vi "Configure Multi Eval Meas Limit OBW.vi"(6 "Limit OBW (40e6)":dbl=40000000.0 format="%^.3e", 7 "Limit OBW Enabled (Value)":i32(ring)=2 items=["Off", "On", "Value"], 8 "error in (no error)":errorcluster, 9 "Bandwidth (5 MHz)":T1=5 items=["5 MHz"=5, "10 MHz"=10, "15 MHz"=15, "20 MHz"=20, "25 MHz"=25, "30 MHz"=30, "40 MHz"=40, "50 MHz"=50, "60 MHz"=60, "80 MHz"=80, "90 MHz"=90, "100 MHz"=100], 10 "Instance (1)":T2=1, 11 "VISA resource name":refnum<visa-resource-name>) -> (0 "error out":errorcluster, 3 "VISA resource name out":refnum<visa-resource-name>)   [LabVIEW 2020, in "Rohde&Schwarz CMWXP NR FR1 Measurement.lvlib"]
doc: "Defines an upper limit for the occupied bandwidth, depending on the channel bandwidth (for NR SA).\n\nAttributes:\nRSCMWXPNRFR1M_ATTR_MULTI_EVAL_MEAS_LIMIT_OBW_ENABLED\nRSCMWXPNRFR1M_ATTR_MULTI_EVAL_MEAS_LIMIT_OBW\n\nRemote-control command:\nCONFigure:NRSub:MEAS<i>:MEValuation:LIMit:SEMask:OBWLimit:CBANdwidth<bw>"
uses:
  <instrlib>/Rohde&Schwarz CMWXP NR FR1 Measurement/Rohde&Schwarz CMWXP NR FR1 Measurement.lvlib
  <instrlib>/Rohde&Schwarz CMWXP NR FR1 Measurement/Private/_Instance.ctl
  <instrlib>/Rohde&Schwarz CMWXP NR FR1 Measurement/Private/_Bandwidth.ctl
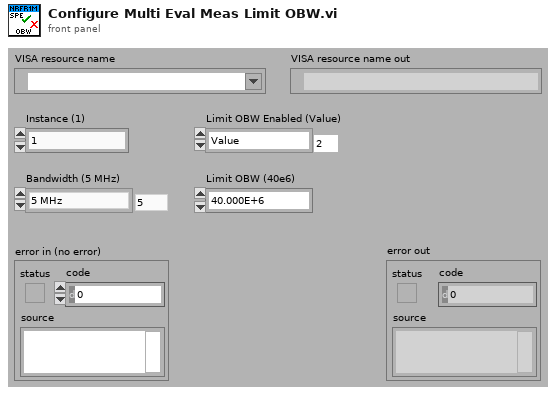
[diagram p1: front panel]
types:
  T1 = typedef "Rohde&Schwarz CMWXP NR FR1 Measurement.lvlib/_Bandwidth.ctl" = i32
  T2 = typedef "Rohde&Schwarz CMWXP NR FR1 Measurement.lvlib/_Instance.ctl" = i32
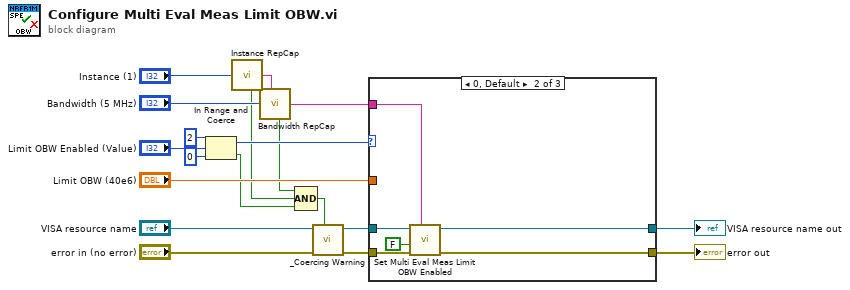
[diagram p0: block diagram]
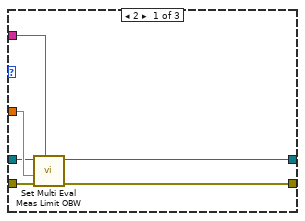
[diagram p2: hidden frame]
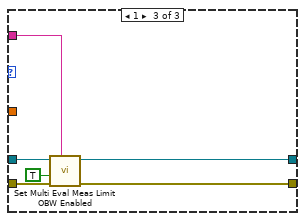
[diagram p3: hidden frame]
diagram:
  n1 = In Range and Coerce(upper limit=2, x="Limit OBW Enabled (Value)", lower limit=0) -> (coerced(x)=w5:i32, In Range?=w4:bool)
  n2 = call <instrlib>:"Instance RepCap.vi"("Instance In"="Instance (1)") -> ("In Range?"=w2:bool, "RepCap Identifier Out"=w15:string)  [unwired: 1 in]
  n3 = call <instrlib>:"Bandwidth RepCap.vi"("Bandwidth (5 MHz)"="Bandwidth (5 MHz)", "RepCap String In (\"\")"=w15) -> ("In Range?"=w3:bool, "RepCap Identifier Out"=w9:string)
  n4 = Compound Arithmetic op=AND(w3, w2, w4) -> (w1:bool)
  n5 = call <instrlib>:"_Coercing Warning.vi"("In Range?"=w1, "error in (no error)"="error in (no error)", "VISA resource name"="VISA resource name") -> ("error out"=w11:errorcluster, "VISA resource name out"=w10:refnum<visa-resource-name>)  [unwired: 7 in]
  n6 = case shown="0, Default" w5 {
    tunnel: [w25 w29 w35] -> w19
    tunnel: [w24 w28 w34] -> w18
    tunnel: "Limit OBW (40e6)" -> [w23 _ _]
    tunnel: w11 -> [w22 w26 w32]
    tunnel: w10 -> [w21 w27 w33]
    tunnel: w9 -> [w20 w31 w37]
    frame 2 {
      n7 = call "Set Multi Eval Meas Limit OBW"("Repeated Capabilities"=w20, "error in (no error)"=w22, "Multi Eval Meas Limit OBW (0.0)"=w23, "instrument handle"=w21) -> ("error out"=w25:errorcluster, "instrument handle out"=w24:refnum<visa-resource-name>)  [unwired: 6 in]
    }
    frame 0, Default {
      n8 = call "Set Multi Eval Meas Limit OBW Enabled"("Repeated Capabilities"=w31, "error in (no error)"=w26, "Multi Eval Meas Limit OBW Enabled (OFF)"=FALSE, "instrument handle"=w27) -> ("error out"=w29:errorcluster, "instrument handle out"=w28:refnum<visa-resource-name>)  [unwired: 6 in]
    }
    frame 1 {
      n9 = call "Set Multi Eval Meas Limit OBW Enabled"("Repeated Capabilities"=w37, "error in (no error)"=w32, "Multi Eval Meas Limit OBW Enabled (OFF)"=TRUE, "instrument handle"=w33) -> ("error out"=w35:errorcluster, "instrument handle out"=w34:refnum<visa-resource-name>)  [unwired: 6 in]
    }
  }
  "error out" <- w19
  "VISA resource name out" <- w18
